vi "lvssh2_userauth_keyboard_interactive_response_function_handler_64.vi"(4 "lvssh2_userauth_keyboard_interactive_response_function":refnum<vi>, 5 "Event Data":T1, 6 "User Event Ref":refnum<user-event>, 7 "Event Common Data":T3 {"Event Source" items=["LabVIEW UI"=0, "ActiveX"=1, "User Event"=25]}) -> ()   [LabVIEW 2017, in "libssh2.lvlib"]
uses:
  libssh2.lvlib
  <vilib>/event_ctls.llb/eventsource.ctl
  lvssh2_userauth_keyboard_interactive_response_function_input_args_64.ctl
  lvssh2_userauth_keyboard_interactive_prompt.ctl
  lvssh2_extensions_64.dll
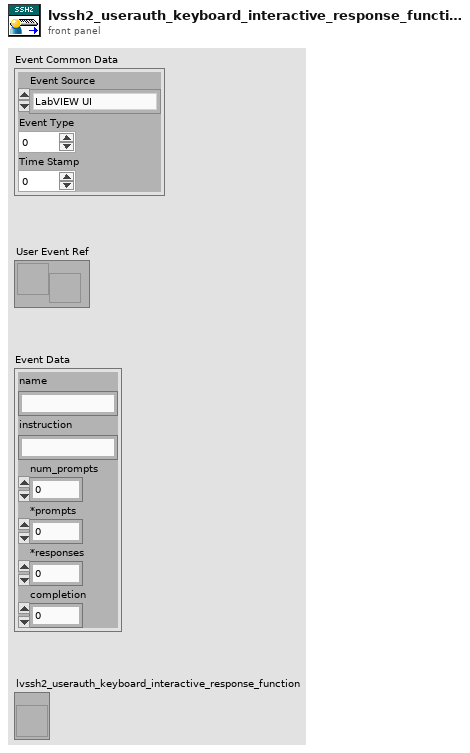
[diagram p1: front panel]
types:
  T1 = typedef "libssh2.lvlib/lvssh2_userauth_keyboard_interactive_response_function_input_args_64.ctl" = cluster{"name":string, "instruction":string, "num_prompts":i32, "*prompts":u64, "*responses":u64, "completion":u64}
  T2 = typedef "eventsource.ctl" = u32
  T3 = cluster{"Event Source":T2, "Event Type":u32, "Time Stamp":u32}
  T4 = typedef "libssh2.lvlib/lvssh2_userauth_keyboard_interactive_prompt.ctl" = cluster{"text":string, "echo":bool}
  T5 = cluster{"text":u64, "length":u64, "echo":u8, "padding-1":u8, "padding-2":u16, "padding-3":u32}
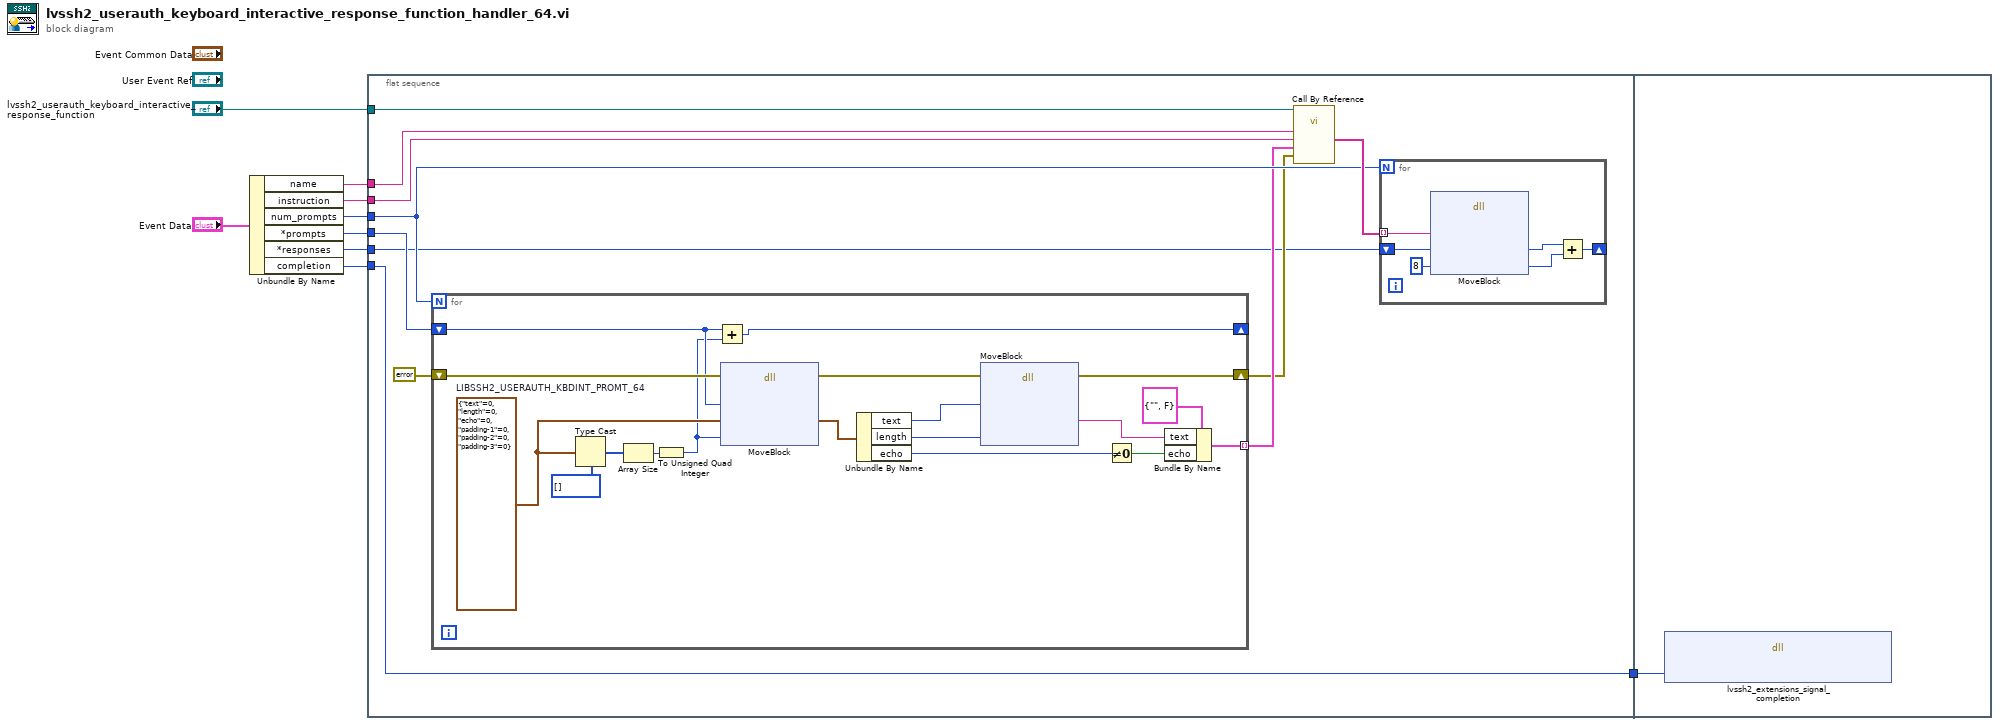
[diagram p0: block diagram]
diagram:
  n1 = Unbundle By Name("Event Data") -> ("name"=w7:string, "instruction"=w6:string, "num_prompts"=w5:i32, "*prompts"=w4:u64, "*responses"=w3:u64, "completion"=w1:u64)
  n2 = flat-sequence {
    tunnel: "lvssh2_userauth_keyboard_interactive_response_function" -> [w20]
    tunnel: w7 -> [w19]
    tunnel: w6 -> [w18]
    tunnel: w5 -> [w16]
    tunnel: w4 -> [w15]
    tunnel: w3 -> [w11]
    tunnel: [w10] -> w2
    tunnel: w1 -> [w10]
    tunnel: w2 -> [w45]
    frame #0 {
      n3 = for {
        N: w16 -> [_]
        tunnel: [w35] -> w14 mode=indexing
        shift-right: [w34] -> _
        shift-left: w15 -> [w31]
        shift-right: [w33] -> w13
        shift-left: errorcluster {"status"=FALSE, "code"=0, "source"=""} ("error out") -> [w32]
        w44 = T5 {"text"=0, "length"=0, "echo"=0, "padding-1"=0, "padding-2"=0, "padding-3"=0}  # LIBSSH2_USERAUTH_KBDINT_PROMT_64
        n4 = Type Cast(type=u8[] [], x=w44) -> (*(type *) &x=w42:u8[])
        n5 = Array Size(array=w42) -> (size(s)=w30:i32)
        n6 = To Unsigned Quad Integer(1:w30) -> (0:w29:u64)
        n7 = Add(x=w31, y=w29) -> (x+y=w34:u64)
        n8 = dll-call lib="LabVIEW" fn="MoveBlock"(error in=w32, "ps"=w31, "pd"=w44, "size"=w29) -> (error out=w41:errorcluster, "pd"=w40:T5)  [unwired: 5 in, 1 out]
        n9 = Unbundle By Name(w40) -> ("text"=w39:u64, "length"=w28:u64, "echo"=w37:u8)
        n10 = dll-call lib="LabVIEW" fn="MoveBlock"(error in=w41, "ps"=w39, "size"=w28) -> (error out=w33:errorcluster, "pd"=w27:string)  [unwired: 6 in, 1 out]
        n11 = Not Equal To 0?(x=w37) -> (x != 0?=w36:bool)
        n12 = Bundle By Name(cluster=T4 {"text"="", "echo"=FALSE} ("prompt"), "text"=w27, "echo"=w36) -> (w35:T4)
      }
      n13 = call-by-ref "?"(reference=w20, "error in (no error)"=w13, "prompts"=w14, "instruction"=w18, "name"=w19) -> ("responses"=w17:string[])  [unwired: 7 in, 3 out]
      n14 = for {
        N: w16 -> [_]
        tunnel: w17 -> [w24] mode=indexing
        shift-right: [w22] -> _
        shift-left: w11 -> [w25]
        n15 = dll-call lib="LabVIEW" fn="MoveBlock"("ps"=w24, "pd"=w25, "size"=u64 8) -> ("pd"=w23:u64, "size"=w21:u64)  [unwired: 5 in, 2 out]
        n16 = Add(x=w23, y=w21) -> (x+y=w22:u64)
      }
    }
    frame #1 {
      n17 = dll-call lib="C:/Users/pasca/Projects/Home/lvssh2/libssh2/lvssh2_extensions**.*" fn="lvssh2_extensions_signal_completion"("completion"=w45) -> ()  [unwired: 5 in, 2 out]
    }
  }
